vi "Parse Config to Queue.vi"(6 "compatible?":bool, 8 "error in":errorcluster, 11 "queue in":T1) -> (0 "error out":errorcluster, 3 "queue out":T1)   [LabVIEW 2010, in "NI_LVConfig.lvlib"]
uses:
  NI_LVConfig.lvlib
  Config Queue.ctl
  Config Data.ctl
  Section.ctl
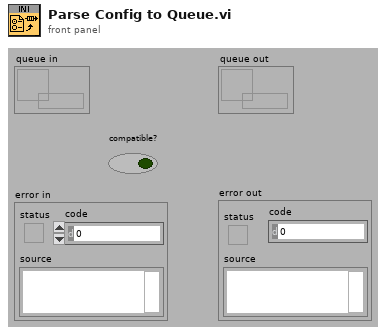
[diagram p1: front panel]
types:
  T1 = typedef "NI_LVConfig.lvlib/Config Queue.ctl" = refnum<queue>
  T2 = typedef "NI_LVConfig.lvlib/Config Data.ctl" = cluster{"sections":T3[], "path":path, "dirty":bool}
  T3 = typedef "NI_LVConfig.lvlib/Section.ctl" = cluster{"name":string, "comment":string, "kvc":string[][]}
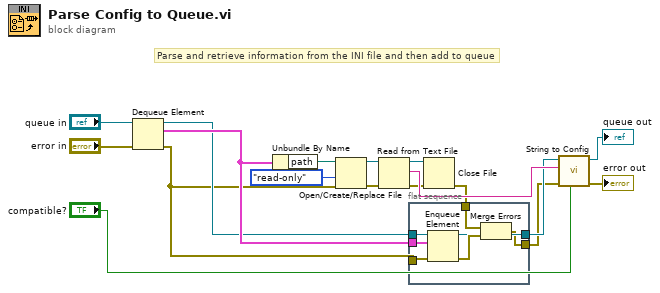
[diagram p0: block diagram]
diagram:
  # "Parse and retrieve information from the INI file and then add to queue"
  n1 = Dequeue Element(queue="queue in", error in (no error)="error in") -> (queue out=w6:T1, element=w7:T2, error out=w4:errorcluster)  [unwired: 1 in, 1 out]
  n2 = Unbundle By Name(w7) -> ("path"=w16:path)
  n3 = Open/Create/Replace File(file path (use dialog)=w16, error in=w4, access (0:read/write)=enum16{"read/write", "read-only", "write-only"}."read-only") -> (refnum out=w14:refnum<file>, error out=w13:errorcluster)  [unwired: 4 out]
  n4 = Read from Text File(file (use dialog)=w14, error in=w13) -> (refnum out=w11:refnum<file>, text=w15:string, error out=w10:errorcluster)  [unwired: 3 out]
  n5 = flat-sequence {
    tunnel: w7 -> [w24]
    tunnel: w6 -> [w23]
    tunnel: [w22] -> w5
    tunnel: w4 -> [w21]
    tunnel: w2 -> [w20]
    tunnel: [w19] -> w1
    frame #0 {
      n6 = Enqueue Element(queue=w23, element=w24, error in (no error)=w21) -> (queue out=w22:T1, error out=w25:errorcluster)  [unwired: 1 in, 1 out]
      n7 = Merge Errors(w20, w25) -> (w19:errorcluster)
    }
  }
  n8 = Close File(refnum=w11, error in=w10) -> (error out=w2:errorcluster)  [unwired: 1 out]
  n9 = call "String to Config.vi"("compatible?"="compatible?", "error in (no error)"=w1, "string input"=w15, "queue in"=w5) -> ("error out"=→"error out":errorcluster, "queue out"=→"queue out":T1)  [unwired: 6 out]
